vi "Write classes.vi"(8 "error in (no error)":errorcluster, 10 "classes":T1, 11 "Channel in":refnum<class "Channel.lvclass">) -> (0 "error out":errorcluster, 3 "Channel out":refnum<class "Channel.lvclass">)   [LabVIEW 2018, in "Channel.lvclass"]
uses:
  Channel.lvclass
  State Machine/State Machine.lvclass
  RxTx/RxTx.lvclass
  Camera/Camera.lvclass
  Request/Request.lvclass
  Channel.lvclass/Channel.ctl
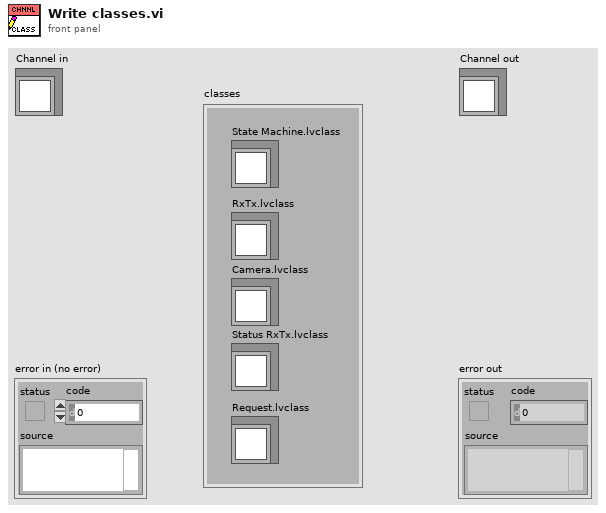
[diagram p1: front panel]
types:
  T1 = cluster{"State Machine.lvclass":refnum<class "State Machine.lvclass">, "RxTx.lvclass":refnum<class "RxTx.lvclass">, "Camera.lvclass":refnum<class "Camera.lvclass">, "Status RxTx.lvclass":refnum<class "RxTx.lvclass">, "Request.lvclass":refnum<class "Request.lvclass">}
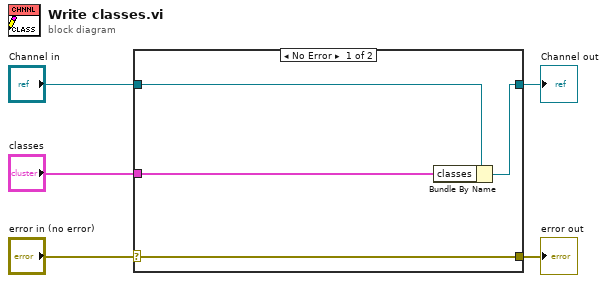
[diagram p0: block diagram]
diagram:
  n1 = case shown="No Error" "error in (no error)" {
    selector: "error in (no error)" -> [w9 w10]
    tunnel: [w9 w10] -> w4
    tunnel: [w7 w11] -> w2
    tunnel: "Channel in" -> [w8 w11]
    tunnel: "classes" -> [w6 _]
    frame No Error {
      n2 = Bundle By Name(cluster=w8, "classes"=w6) -> (w7:refnum<class "Channel.lvclass">)
    }
    frame Error {
    }
  }
  "error out" <- w4
  "Channel out" <- w2
